vi "BooleanCaseString.vi"(5 "selector string":string) -> (1 "Default":bool, 4 "case":string)   [LabVIEW 2014, in "Raspberry Pi Compatible Compiler for LabVIEW.lvlib" / "CaseStructure.lvclass"]
uses:
  CaseStructure.lvclass
  Python/Parsing/ListTypesTD.ctl
  Python/Parsing/Python Functions.lvlib
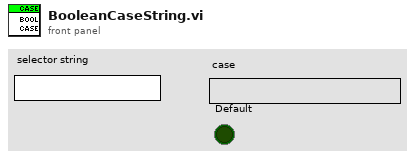
[diagram p1: front panel]
types:
  T1 = typedef "Raspberry Pi Compatible Compiler for LabVIEW.lvlib/Python Functions.lvlib/ListTypesTD.ctl" = enum16{"list", "tuple", "parameter list", "output list", "return values"}
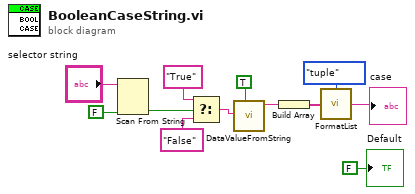
[diagram p0: block diagram]
diagram:
  n1 = Scan From String(input string="selector string", default 1=FALSE) -> (output 1=w4:bool)  [unwired: 3 in, 3 out]
  n2 = Select(t="True", s=w4, f="False") -> (s? t:f=w1:string)
  n3 = call "DataValueFromString.vi"("Type"=TRUE, "value"=w1) -> ("value"=w9:string)  [unwired: 7 in]
  n4 = Build Array(w9) -> (w8:string[])
  n5 = call "FormatList.vi"("values"=w8, "type"=ListTypesTD."tuple") -> ("python object"=→"case":string)
  "Default" <- FALSE ("Default")
